vi "UI_ExamplesubVI.vi"() -> ()   [LabVIEW 2018]
panel:
  out "NewVal":dbl
  in  "UI_Num2":dbl
  in  "UI_Num1":dbl
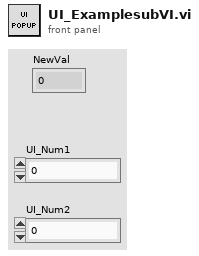
[diagram p1: front panel]
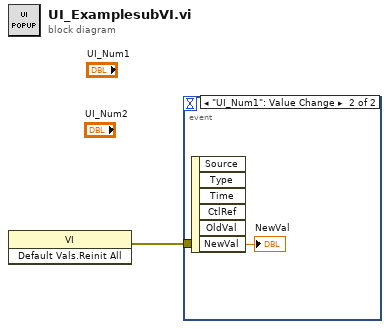
[diagram p0: block diagram]
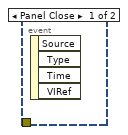
[diagram p2: hidden frame]
diagram:
  n1 = invoke class="VI" method="Default Vals.Reinit All"() -> (error out=w1:errorcluster)  [unwired: 3 in, 2 out]
  n2 = event shown="[1] \"UI_Num1\": Value Change" {
    selector: _ -> [_ _]
    dyn-events: _ -> [_ _]
    timeout: _ -> [_ _]
    tunnel: w1 -> [_ _]
    event Panel Close {
      n3 = event-data() -> ()  [unwired: 1 in, 4 out]
    }
    event "UI_Num1": Value Change {
      n4 = event-data() -> ("NewVal"=→"NewVal":dbl)  [unwired: 1 in, 5 out]
    }
  }
